vi "CRC32.vi"(11 "Data":string) -> (3 "CRC32Value":u32 format="%x")   [LabVIEW 2013]
doc: "Standard CRC32 calculator curtesy of Internet LabView community member DGardner.\n\nVI icon curtesy of our programmer Rachel Gardner (no relation to the aforementioned programmer)."
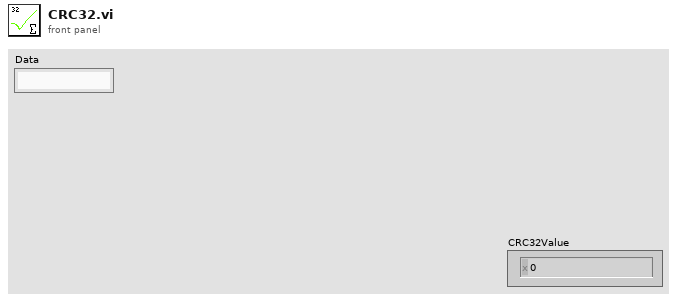
[diagram p1: front panel]
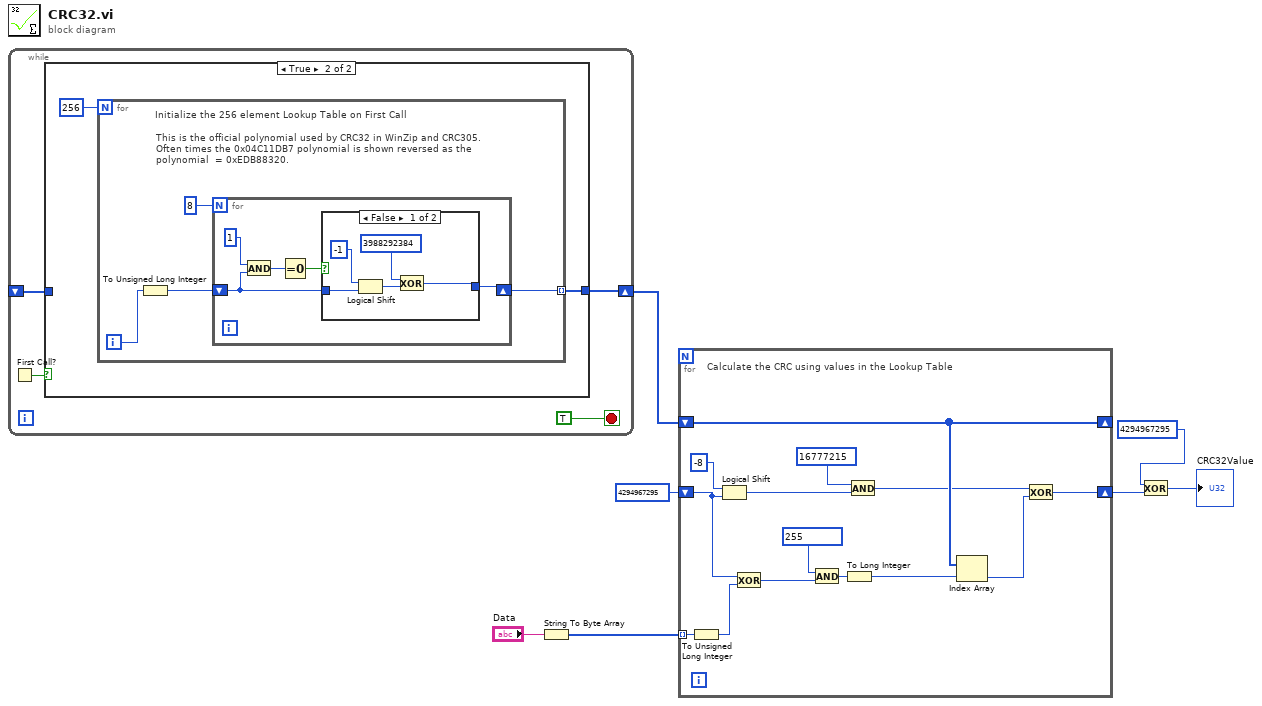
[diagram p0: block diagram]
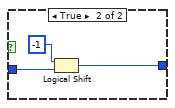
[diagram p3: hidden frame]
diagram:
  n1 = while {
    shift-right: [w10] -> w3
    shift-left: _ -> [w9]
    stop <- TRUE stop-if-true
    n2 = First Call?() -> (First Call?: T/F=w11:bool)
    n3 = case shown="True" w11 {
      tunnel: [w12 w13] -> w10
      tunnel: w9 -> [w12 _]
      frame False {
      }
      frame True {
        n4 = for {
          N: 256 -> [_]
          tunnel: [w17] -> w13 mode=indexing
          i -> [w16]
          # "This is the official polynomial used by CRC32 in WinZip and CRC305.\nOften times the 0x04C11DB7 polynomial is shown reversed as the\npolynomial  = 0xEDB88320."
          # "Initialize the 256 element Lookup Table on First Call"
          n5 = To Unsigned Long Integer(number=w16) -> (unsigned 32bit integer=w15:u32)
          n6 = for {
            N: 8 -> [_]
            shift-right: [w23] -> w17
            shift-left: w15 -> [w22]
            n7 = And(x=u32 1, y=w22) -> (x .and. y?=w21:u32)
            n8 = Equal To 0?(x=w21) -> (x = 0?=w19:bool)
            n9 = case shown="False" w19 {
              tunnel: w22 -> [w28 w31]
              tunnel: [w24 w29] -> w23
              frame False {
                n10 = Logical Shift(y=-1, x=w28) -> (x << y=w26:u32)
                n11 = Exclusive Or(1:w26, 2:u32 3988292384) -> (0:w24:u32)
              }
              frame True {
                n12 = Logical Shift(y=-1, x=w31) -> (x << y=w29:u32)
              }
            }
          }
        }
      }
    }
  }
  n13 = String To Byte Array(string="Data") -> (unsigned byte array=w7:u8[])
  n14 = for {
    tunnel: w7 -> [w45] mode=indexing
    shift-right: [w38] -> w6
    shift-left: u32 4294967295 -> [w34]
    shift-right: [w37] -> _
    shift-left: w3 -> [w37]
    # "Calculate the CRC using values in the Lookup Table"
    n15 = To Unsigned Long Integer(number=w45) -> (unsigned 32bit integer=w44:u32)
    n16 = Logical Shift(y=-8, x=w34) -> (x << y=w39:u32)
    n17 = Exclusive Or(1:w44, 2:w34) -> (0:w42:u32)
    n18 = And(x=u32 255, y=w42) -> (x .and. y?=w33:u32)
    n19 = To Long Integer(number=w33) -> (32bit integer=w41:i32)
    n20 = And(x=u32 16777215, y=w39) -> (x .and. y?=w36:u32)
    n21 = Index Array "Index Array"(array=w37, index=w41) -> (element=w40:u32)
    n22 = Exclusive Or(1:w40, 2:w36) -> (0:w38:u32)
  }
  n23 = Exclusive Or(1:w6, 2:u32 4294967295) -> (0:→"CRC32Value":u32)
